vi "Remove Project.vi"(8 "error in (no error)":errorcluster, 10 "Project Name":string, 11 "Projects in":refnum<class "Projects.lvclass">) -> (0 "error out":errorcluster, 2 "Deleted?":bool, 3 "Projects out":refnum<class "Projects.lvclass">)   [LabVIEW 2020, in "Projects.lvclass"]
doc: "Removes (Deletes) the named project from the Map. This method will return a True to the Deleted? indicator only if the Project Name is present and the project was removed from the Map.\n\n03/2025 Erich Schlieper"
uses:
  Projects.lvclass
  Projects.lvclass/Projects.ctl
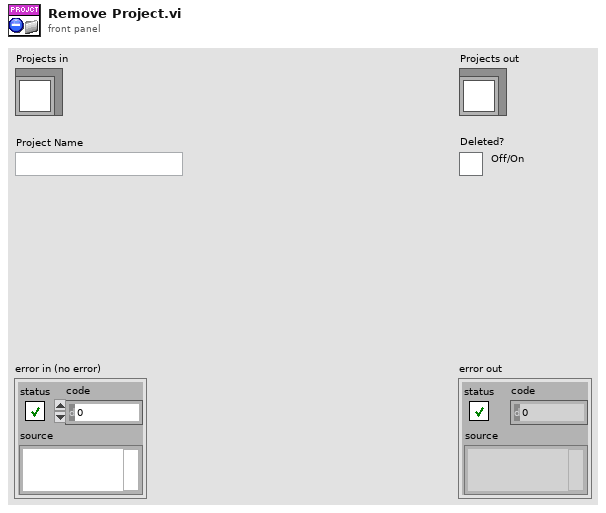
[diagram p1: front panel]
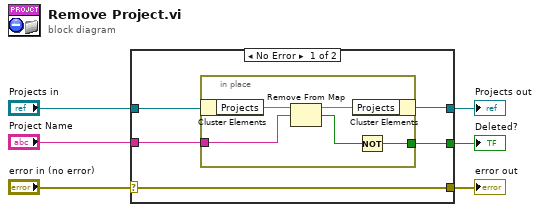
[diagram p0: block diagram]
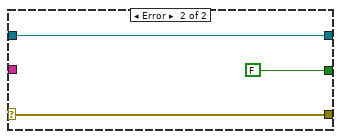
[diagram p2: hidden frame]
diagram:
  n1 = case shown="No Error" "error in (no error)" {
    selector: "error in (no error)" -> [w10 w19]
    tunnel: [w10 w19] -> w5
    tunnel: [w9 w18] -> w3
    tunnel: "Projects in" -> [w11 w18]
    tunnel: "Project Name" -> [w8 _]
    tunnel: [w7 FALSE] -> w1
    frame No Error {
      n2 = in-place {
        in-place-border: w8 -> [w14]
        in-place-border: [w12] -> w7
        n3 = in-place-cluster #1(w11) -> ("Projects"=w16:map{string, set{string}})
        n4 = Remove From Map(10:w14, 11:w16) -> (2:w13:bool, 3:w15:map{string, set{string}})  [unwired: 1 out]
        n5 = in-place-cluster #1("Projects"=w15) -> (w9:refnum<class "Projects.lvclass">)
        n6 = Not(x=w13) -> (.not. x?=w12:bool)
      }
    }
    frame Error {
    }
  }
  "error out" <- w5
  "Projects out" <- w3
  "Deleted?" <- w1
